vi "Process combined pos.vi"(9 "Pos ref":T1, 10 "Gyro data":T2, 11 "Acc data":cluster{"Acc X":i16, "Acc Y":i16, "Acc Z":i16}) -> (0 "Y tg":dbl, 1 "Y processed":dbl, 2 "X processed":dbl, 3 "X tg":dbl)   [LabVIEW 2017]
uses:
  <userlib>/_MGI/Numeric/Coercion/MGI Radians to Degrees/MGI Radians to Degrees DBL.vi
panel:
  out "XY Graph - Dark":cluster{"X":dbl, "Y":dbl}[](graph) caption="XY Graph - dark"
  out "X sin":dbl format="%.2f"
  out "Y deg":dbl format="%.2f"
  out "X deg":dbl format="%.2f"
  out "sqrt(x)":dbl format="%#.1f"
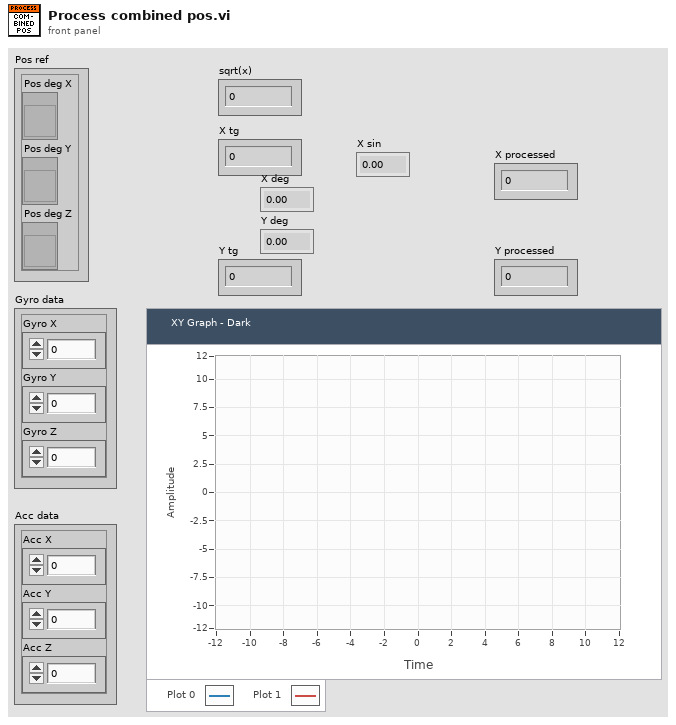
[diagram p1: front panel]
types:
  T1 = cluster{"Pos deg X":refnum<vi>, "Pos deg Y":refnum<vi>, "Pos deg Z":refnum<vi>}
  T2 = cluster{"Gyro X":i16, "Gyro Y":i16, "Gyro Z":i16}
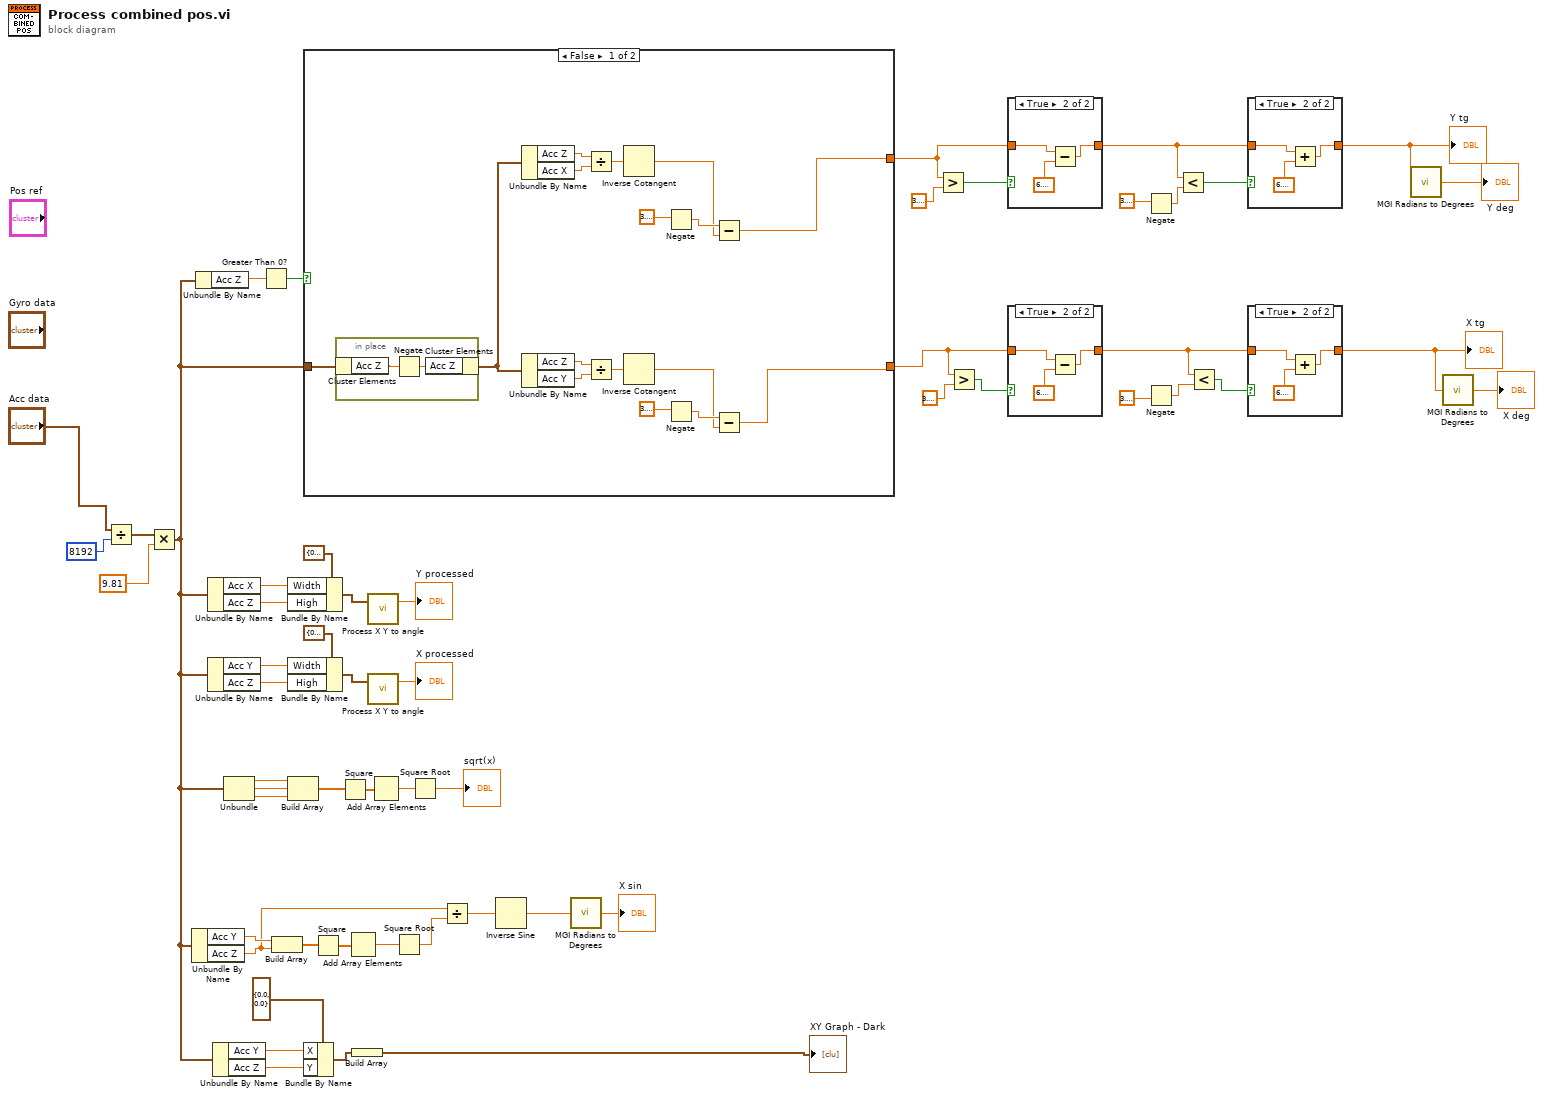
[diagram p0: block diagram]
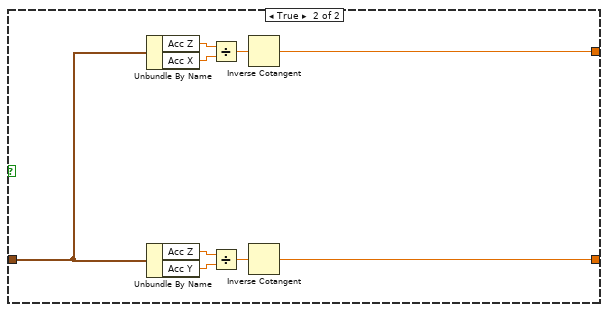
[diagram p2: hidden frame]
diagram:
  n1 = Divide(x="Acc data", y=8192) -> (x/y=w54:cluster{"Acc X":dbl, "Acc Y":dbl, "Acc Z":dbl})
  n2 = Multiply(x=w54, y=9.81) -> (x*y=w1:cluster{"Acc X":dbl, "Acc Y":dbl, "Acc Z":dbl})
  n3 = Unbundle By Name(w1) -> ("Acc Y"=w21:dbl, "Acc Z"=w12:dbl)
  n4 = Unbundle By Name(w1) -> ("Acc Z"=w27:dbl)
  n5 = Unbundle By Name(w1) -> ("Acc X"=w10:dbl, "Acc Z"=w9:dbl)
  n6 = Unbundle By Name(w1) -> ("Acc Y"=w3:dbl, "Acc Z"=w4:dbl)
  n7 = Unbundle By Name(w1) -> ("Acc Y"=w16:dbl, "Acc Z"=w15:dbl)
  n8 = Unbundle(w1) -> ("Acc X"=w52:dbl, "Acc Y"=w51:dbl, "Acc Z"=w50:dbl)
  n9 = Greater Than 0?(x=w27) -> (x > 0?=w26:bool)
  n10 = Build Array(w21, w12) -> (w23:dbl[])
  n11 = Bundle By Name(cluster=cluster{"Width":dbl, "High":dbl} {"Width"=0.0, "High"=0.0} ("Point position"), "Width"=w10, "High"=w9) -> (w8:cluster{"Width":dbl, "High":dbl})
  n12 = Bundle By Name(cluster=cluster{"Width":dbl, "High":dbl} {"Width"=0.0, "High"=0.0} ("Point position"), "Width"=w3, "High"=w4) -> (w5:cluster{"Width":dbl, "High":dbl})
  n13 = Build Array(w52, w51, w50) -> (w49:dbl[])
  n14 = case shown="False" w26 {
    tunnel: w1 -> [w66 w75]
    tunnel: [w57 w77] -> w41
    tunnel: [w61 w76] -> w39
    frame False {
      n15 = in-place {
        n16 = in-place-cluster #1(w66) -> ("Acc Z"=w74:dbl)
        n17 = Negate(x=w74) -> (-x=w73:dbl)
        n18 = in-place-cluster #1("Acc Z"=w73) -> (w65:cluster{"Acc X":dbl, "Acc Y":dbl, "Acc Z":dbl})
      }
      n19 = Unbundle By Name(w65) -> ("Acc Z"=w68:dbl, "Acc X"=w70:dbl)
      n20 = Unbundle By Name(w65) -> ("Acc Z"=w67:dbl, "Acc Y"=w71:dbl)
      n21 = Divide(x=w68, y=w70) -> (x/y=w69:dbl)
      n22 = Divide(x=w67, y=w71) -> (x/y=w72:dbl)
      n23 = Inverse Cotangent(1:w69) -> (0:w58:dbl)
      n24 = Inverse Cotangent(1:w72) -> (0:w62:dbl)
      n25 = Negate(x=3.141592653589793) -> (-x=w60:dbl)
      n26 = Negate(x=3.141592653589793) -> (-x=w63:dbl)
      n27 = Subtract(x=w60, y=w58) -> (x-y=w57:dbl)
      n28 = Subtract(x=w63, y=w62) -> (x-y=w61:dbl)
    }
    frame True {
      n29 = Unbundle By Name(w75) -> ("Acc Z"=w79:dbl, "Acc X"=w81:dbl)
      n30 = Unbundle By Name(w75) -> ("Acc Z"=w78:dbl, "Acc Y"=w82:dbl)
      n31 = Divide(x=w79, y=w81) -> (x/y=w80:dbl)
      n32 = Divide(x=w78, y=w82) -> (x/y=w83:dbl)
      n33 = Inverse Cotangent(1:w80) -> (0:w77:dbl)
      n34 = Inverse Cotangent(1:w83) -> (0:w76:dbl)
    }
  }
  n35 = Bundle By Name(cluster=cluster{"X":dbl, "Y":dbl} {"X"=0.0, "Y"=0.0}, "X"=w16, "Y"=w15) -> (w14:cluster{"X":dbl, "Y":dbl})
  n36 = Square(x=w23) -> (x^2=w24:dbl[])
  n37 = Square(x=w49) -> (x^2=w48:dbl[])
  n38 = Add Array Elements(numeric array=w24) -> (sum=w25:dbl)
  n39 = Build Array(w14) -> (→"XY Graph - Dark":cluster{"X":dbl, "Y":dbl}[])
  n40 = call "Process X Y to angle.vi"("Point position"=w8) -> ("Angle (rad)"=→"Y processed":dbl)  [unwired: 2 in]
  n41 = call "Process X Y to angle.vi"("Point position"=w5) -> ("Angle (rad)"=→"X processed":dbl)  [unwired: 2 in]
  n42 = Add Array Elements(numeric array=w48) -> (sum=w47:dbl)
  n43 = Square Root(x=w25) -> (sqrt(x)=w22:dbl)
  n44 = Square Root(x=w47) -> (sqrt(x)=→"sqrt(x)":dbl)
  n45 = Divide(x=w12, y=w22) -> (x/y=w20:dbl)
  n46 = Inverse Sine(1:w20) -> (0:w19:dbl)
  n47 = call-poly <userlib>:"MGI Radians to Degrees.vi"("Radians"=w19) -> ("Degrees"=→"X sin":dbl)
  n48 = Greater?(x=w41, y=3.141592653589793) -> (0:w42:bool)
  n49 = Greater?(x=w39, y=3.141592653589793) -> (0:w38:bool)
  n50 = case shown="True" w42 {
    tunnel: w41 -> [w84 w87]
    tunnel: [w84 w85] -> w34
    frame False {
    }
    frame True {
      n51 = Subtract(x=w87, y=6.283185307179586) -> (x-y=w85:dbl)
    }
  }
  n52 = case shown="True" w38 {
    tunnel: w39 -> [w88 w91]
    tunnel: [w88 w89] -> w35
    frame False {
    }
    frame True {
      n53 = Subtract(x=w91, y=6.283185307179586) -> (x-y=w89:dbl)
    }
  }
  n54 = Negate(x=3.141592653589793) -> (-x=w28:dbl)
  n55 = Negate(x=3.141592653589793) -> (-x=w30:dbl)
  n56 = Less?(x=w34, y=w28) -> (x < y?=w36:bool)
  n57 = Less?(x=w35, y=w30) -> (x < y?=w37:bool)
  n58 = case shown="True" w36 {
    tunnel: w34 -> [w92 w95]
    tunnel: [w92 w93] -> w33
    frame False {
    }
    frame True {
      n59 = Add(x=w95, y=6.283185307179586) -> (x+y=w93:dbl)
    }
  }
  "Y tg" <- w33
  n60 = case shown="True" w37 {
    tunnel: w35 -> [w96 w99]
    tunnel: [w96 w97] -> w32
    frame False {
    }
    frame True {
      n61 = Add(x=w99, y=6.283185307179586) -> (x+y=w97:dbl)
    }
  }
  "X tg" <- w32
  n62 = call-poly <userlib>:"MGI Radians to Degrees.vi"("Radians"=w33) -> ("Degrees"=→"Y deg":dbl)
  n63 = call-poly <userlib>:"MGI Radians to Degrees.vi"("Radians"=w32) -> ("Degrees"=→"X deg":dbl)
